vi "set settings from string.vi"(8 "error constant":errorcluster, 10 "String":string, 11 "VI in":refnum<vi>) -> (0 "error out":errorcluster)   [LabVIEW 2016, in "SaveLoad.lvlib"]
uses:
  SaveLoad.lvlib
  <vilib>/Utility/Data Type/Type Definitions/Data Type.ctl
  <vilib>/Utility/Data Type/NI_Data Type.lvlib
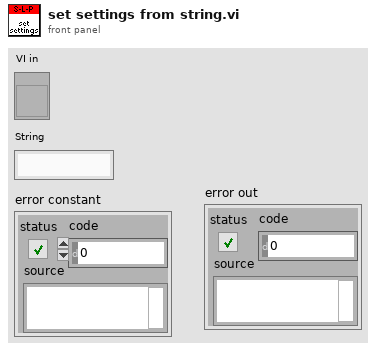
[diagram p1: front panel]
types:
  T1 = typedef "NI_Data Type.lvlib/Data Type.ctl" = enum8{"Invalid Type", "Void", "I8", "I16", "I32", "I64", "U8", "U16", "U32", "U64", "Single Float", "Double Float", "Extended Float", "Single Complex", "Double Complex", "Extended Complex", "Enum U8", "Enum U16", "Enum U32", "Enum U64", "Single Float With Unit", "Double Float With Unit", "Extended Float With Unit", "Single Complex with Unit", "Double Complex with Unit", "Extended Complex with Unit", "Boolean", "String", "Path", "Picture", "Tag", "Array", "Cluster", "Variant", "LV Variant", "Waveform", "Timestamp", "Digital Waveform", "Digital Data", "ExpressData", "Refnum", "External Data", "VI", "Poly VI", "LabVIEW Class Instance", "Fixed Point"}
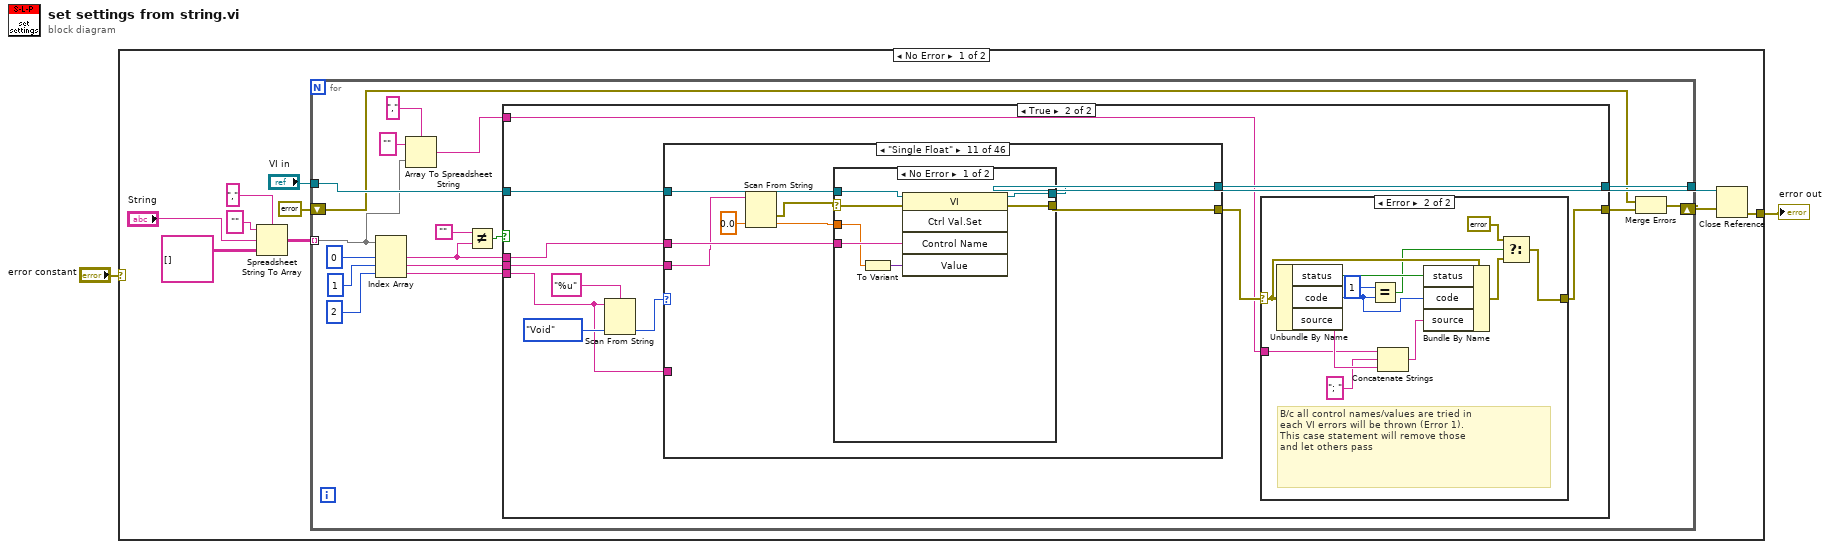
[diagram p0: block diagram]
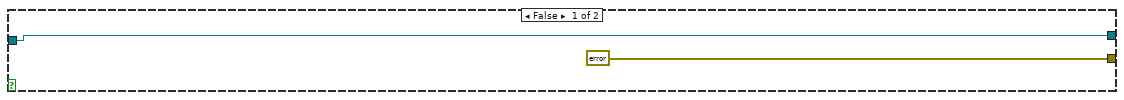
[diagram p2: hidden frame]
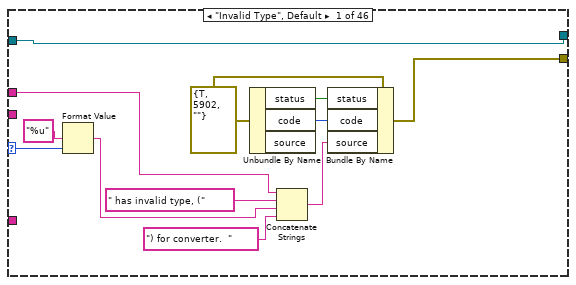
[diagram p4: hidden frame]
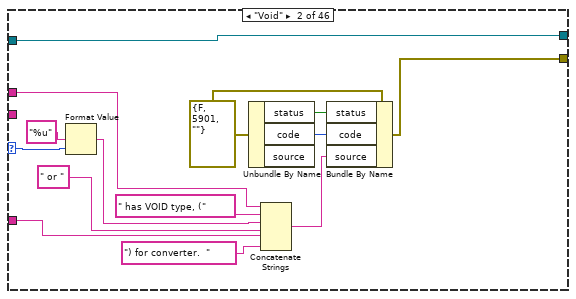
[diagram p5: hidden frame]
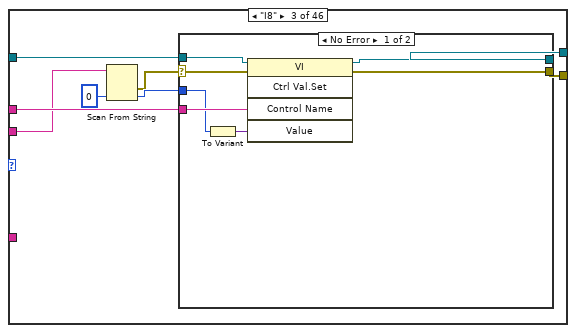
[diagram p6: hidden frame]
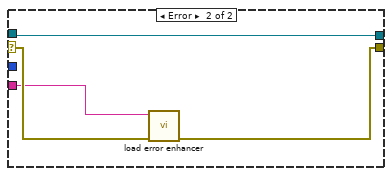
[diagram p7: hidden frame]
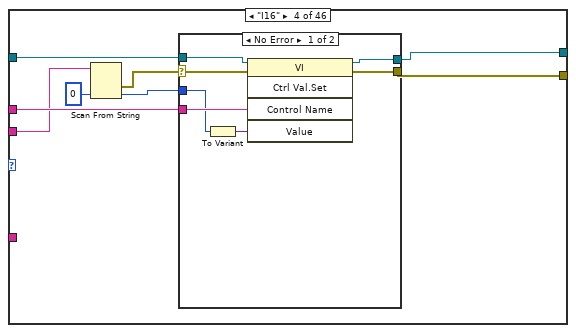
[diagram p8: hidden frame]
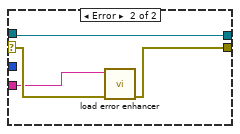
[diagram p9: hidden frame]
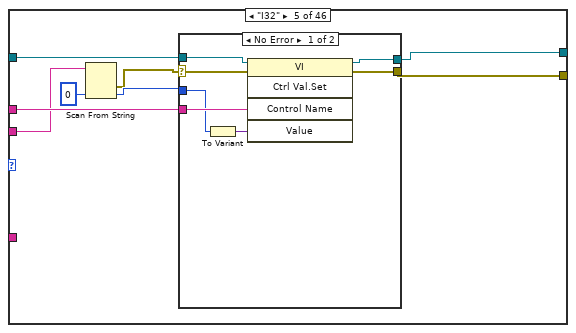
[diagram p10: hidden frame]
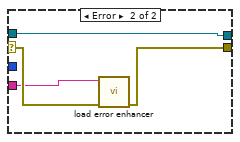
[diagram p11: hidden frame]
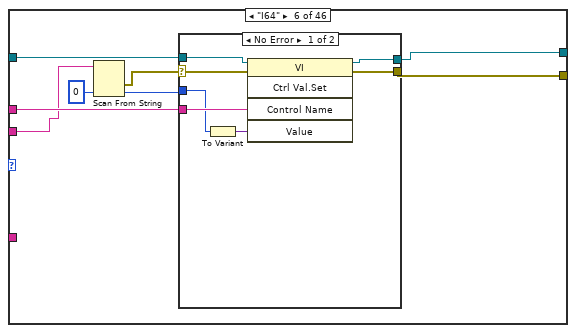
[diagram p12: hidden frame]
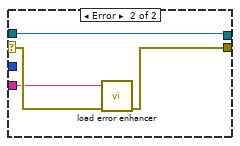
[diagram p13: hidden frame]
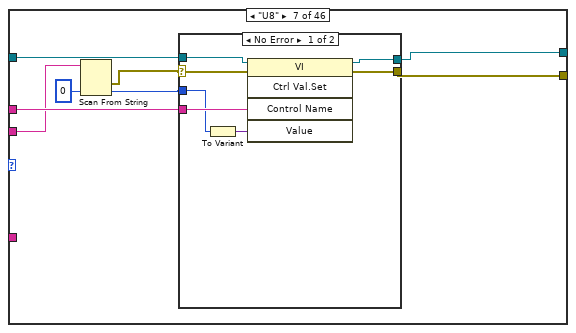
[diagram p14: hidden frame]
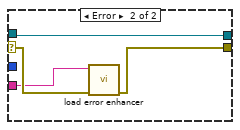
[diagram p15: hidden frame]
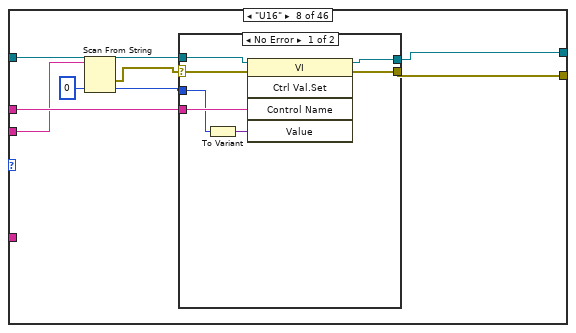
[diagram p16: hidden frame]
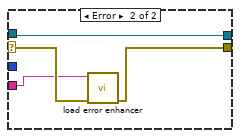
[diagram p17: hidden frame]
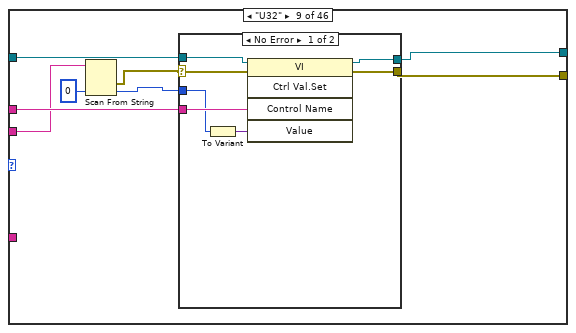
[diagram p18: hidden frame]
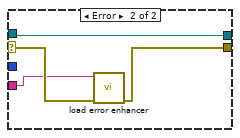
[diagram p19: hidden frame]
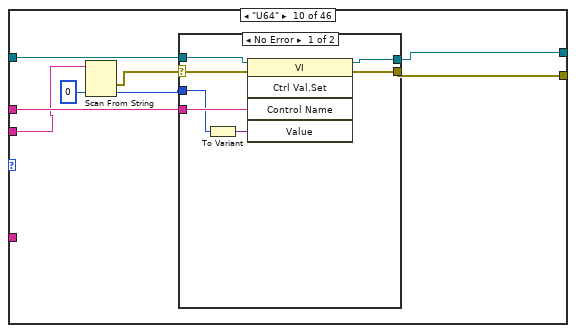
[diagram p20: hidden frame]
diagram:
  n1 = case shown="No Error" "error constant" {
    selector: "error constant" -> [_ w414]
    tunnel: [w12 w414] -> w2
    frame No Error {
      n2 = Spreadsheet String To Array(delimiter (Tab)=",", format string="", spreadsheet string="String", array type (2D Dbl)=string[][] []) -> (array=w8:string[][])
      n3 = for {
        tunnel: w8 -> [w16] mode=indexing
        tunnel: "VI in" -> [w25]
        tunnel: [w24] -> w10
        shift-right: [w21] -> w11
        shift-left: errorcluster {"status"=FALSE, "code"=0, "source"=""} ("error out") -> [w20]
        n4 = Index Array(array=w16, index #1=0 ("index"), index #2=1 ("index"), index #3=2 ("index")) -> (element #1=w18:string, element #2=w26:string, element #3=w22:string)
        n5 = Array To Spreadsheet String(delimiter (Tab)=",", array=w16, 3:"" ("format string")) -> (spreadsheet string=w13:string)
        n6 = Not Equal?(x="", y=w18) -> (x != y?=w17:bool)
        n7 = case shown="True" w17 {
          tunnel: w26 -> [_ w42]
          tunnel: w25 -> [w31 w41]
          tunnel: [w31 w40] -> w24
          tunnel: [errorcluster {"status"=FALSE, "code"=0, "source"=""} ("error out") w32] -> w23
          tunnel: w22 -> [_ w37]
          tunnel: w18 -> [_ w34]
          tunnel: w13 -> [_ w33]
          frame False {
          }
          frame True {
            n8 = Scan From String(format string="%u", input string=w37, default 1=Data_Type."Void" ("Type")) -> (output 1=w39:T1)  [unwired: 2 in, 3 out]
            n9 = case shown="\"Single Float\"" w39 {
              selector: w39 -> [w58 w72 _ _ _ _ _ _ _ _ _ _ _ _ _ _ _ _ _ _ _ _ _ _ _ _ _ _ _ _ _ _ _ _ _ _ _ _ _ _ _ _ _ _ _ _]
              tunnel: w34 -> [w62 w74 w89 w108 w127 w146 w165 w184 w203 w222 w241 w260 w279 w301 w318 w327 _ _ _ _ _ _ _ _ _ _ _ _ _ _ _ _ _ _ _ _ _ _ _ _ _ _ _ _ _ w402]
              tunnel: w42 -> [_ _ w82 w101 w120 w141 w160 w179 w196 w217 w236 w253 w272 w296 w317 w323 _ _ _ _ _ _ _ _ _ _ _ _ _ _ _ _ _ _ _ _ _ _ _ _ _ _ _ _ _ w398]
              tunnel: w41 -> [w67 w81 w88 w107 w126 w145 w164 w183 w202 w221 w240 w259 w278 w300 w316 w320 w338 w340 w342 w344 w346 w348 w350 w352 w354 w356 w358 w360 w362 w364 w366 w368 w370 w372 w374 w376 w378 w380 w382 w384 w386 w388 w390 w392 w394 w401]
              tunnel: [w67 w81 w87 w106 w125 w144 w163 w182 w201 w220 w239 w258 w277 w299 w315 w326 w338 w340 w342 w344 w346 w348 w350 w352 w354 w356 w358 w360 w362 w364 w366 w368 w370 w372 w374 w376 w378 w380 w382 w384 w386 w388 w390 w392 w394 w400] -> w40
              tunnel: [w65 w75 w86 w105 w124 w143 w162 w181 w200 w219 w238 w257 w276 w298 w314 w321 errorcluster {"status"=FALSE, "code"=0, "source"=""} ("error out") errorcluster {"status"=FALSE, "code"=0, "source"=""} ("error out") errorcluster {"status"=FALSE, "code"=0, "source"=""} ("error out") errorcluster {"status"=FALSE, "code"=0, "source"=""} ("error out") errorcluster {"status"=FALSE, "code"=0, "source"=""} ("error out") errorcluster {"status"=FALSE, "code"=0, "source"=""} ("error out") errorcluster {"status"=FALSE, "code"=0, "source"=""} ("error out") errorcluster {"status"=FALSE, "code"=0, "source"=""} ("error out") errorcluster {"status"=FALSE, "code"=0, "source"=""} ("error out") errorcluster {"status"=FALSE, "code"=0, "source"=""} ("error out") errorcluster {"status"=FALSE, "code"=0, "source"=""} ("error out") errorcluster {"status"=FALSE, "code"=0, "source"=""} ("error out") errorcluster {"status"=FALSE, "code"=0, "source"=""} ("error out") errorcluster {"status"=FALSE, "code"=0, "source"=""} ("error out") errorcluster {"status"=FALSE, "code"=0, "source"=""} ("error out") errorcluster {"status"=FALSE, "code"=0, "source"=""} ("error out") errorcluster {"status"=FALSE, "code"=0, "source"=""} ("error out") errorcluster {"status"=FALSE, "code"=0, "source"=""} ("error out") errorcluster {"status"=FALSE, "code"=0, "source"=""} ("error out") errorcluster {"status"=FALSE, "code"=0, "source"=""} ("error out") errorcluster {"status"=FALSE, "code"=0, "source"=""} ("error out") errorcluster {"status"=FALSE, "code"=0, "source"=""} ("error out") errorcluster {"status"=FALSE, "code"=0, "source"=""} ("error out") errorcluster {"status"=FALSE, "code"=0, "source"=""} ("error out") errorcluster {"status"=FALSE, "code"=0, "source"=""} ("error out") errorcluster {"status"=FALSE, "code"=0, "source"=""} ("error out") errorcluster {"status"=FALSE, "code"=0, "source"=""} ("error out") errorcluster {"status"=FALSE, "code"=0, "source"=""} ("error out") errorcluster {"status"=FALSE, "code"=0, "source"=""} ("error out") w399] -> w35
              tunnel: w37 -> [_ w70 _ _ _ _ _ _ _ _ _ _ _ _ _ _ _ _ _ _ _ _ _ _ _ _ _ _ _ _ _ _ _ _ _ _ _ _ _ _ _ _ _ _ _ _]
              frame "Invalid Type", Default {
                w66 = errorcluster {"status"=TRUE, "code"=5902, "source"=""} ("error constant")
                n10 = Format Value(format string="%u", value (0)=w58) -> (output string=w57:string)  [unwired: 1 in]
                n11 = Unbundle By Name(w66) -> ("status"=w64:bool, "code"=w63:i32)  [unwired: 1 out]
                n12 = Concatenate Strings(w62, " has invalid type, (", w57, ") for converter.  " ("string")) -> (w60:string)
                n13 = Bundle By Name(cluster=w66, "status"=w64, "code"=w63, "source"=w60) -> (w65:errorcluster)
              }
              frame "Void" {
                w80 = errorcluster {"status"=FALSE, "code"=5901, "source"=""} ("error constant")
                n14 = Format Value(format string="%u", value (0)=w72) -> (output string=w69:string)  [unwired: 1 in]
                n15 = Unbundle By Name(w80) -> ("status"=w79:bool, "code"=w78:i32)  [unwired: 1 out]
                n16 = Concatenate Strings(w74, " has VOID type, (", w69, " or " ("string"), w70, ") for converter.  " ("string")) -> (w76:string)
                n17 = Bundle By Name(cluster=w80, "status"=w79, "code"=w78, "source"=w76) -> (w75:errorcluster)
              }
              frame "I8" {
                n18 = Scan From String(input string=w82, default 1=i8 0 ("default value 1")) -> (error out=w84:errorcluster, output 1=w85:i8)  [unwired: 3 in, 2 out]
                n19 = case shown="No Error" w84 {
                  selector: w84 -> [w90 w98]
                  tunnel: [w96 w100] -> w87
                  tunnel: [w95 w99] -> w86
                  tunnel: w89 -> [w94 w97]
                  tunnel: w85 -> [w92 _]
                  tunnel: w88 -> [w91 w100]
                  frame No Error {
                    n20 = To Variant(anything=w92) -> (Variant=w93:variant)
                    n21 = invoke class="VI" method="Ctrl Val.Set"(reference=w91, error in=w90, "Control Name"=w94, "Value"=w93) -> (reference out=w96:refnum<vi>, error out=w95:errorcluster)  [unwired: 1 in, 3 out]
                  }
                  frame Error {
                    n22 = call "load error enhancer.vi"("error in (no error)"=w98, "format string"=w97) -> ("error out"=w99:errorcluster)  [unwired: 9 in]
                  }
                }
              }
              frame "I16" {
                n23 = Scan From String(input string=w101, default 1=i16 0 ("default value 1")) -> (error out=w104:errorcluster, output 1=w103:i16)  [unwired: 3 in, 2 out]
                n24 = case shown="No Error" w104 {
                  selector: w104 -> [w109 w118]
                  tunnel: [w115 w119] -> w106
                  tunnel: [w114 w116] -> w105
                  tunnel: w108 -> [w113 w117]
                  tunnel: w103 -> [w111 _]
                  tunnel: w107 -> [w110 w119]
                  frame No Error {
                    n25 = To Variant(anything=w111) -> (Variant=w112:variant)
                    n26 = invoke class="VI" method="Ctrl Val.Set"(reference=w110, error in=w109, "Control Name"=w113, "Value"=w112) -> (reference out=w115:refnum<vi>, error out=w114:errorcluster)  [unwired: 1 in, 3 out]
                  }
                  frame Error {
                    n27 = call "load error enhancer.vi"("error in (no error)"=w118, "format string"=w117) -> ("error out"=w116:errorcluster)  [unwired: 9 in]
                  }
                }
              }
              frame "I32" {
                n28 = Scan From String(input string=w120, default 1=0 ("default value 1")) -> (error out=w121:errorcluster, output 1=w122:i32)  [unwired: 3 in, 2 out]
                n29 = case shown="No Error" w121 {
                  selector: w121 -> [w128 w137]
                  tunnel: [w134 w138] -> w125
                  tunnel: [w133 w135] -> w124
                  tunnel: w127 -> [w132 w136]
                  tunnel: w122 -> [w130 _]
                  tunnel: w126 -> [w129 w138]
                  frame No Error {
                    n30 = To Variant(anything=w130) -> (Variant=w131:variant)
                    n31 = invoke class="VI" method="Ctrl Val.Set"(reference=w129, error in=w128, "Control Name"=w132, "Value"=w131) -> (reference out=w134:refnum<vi>, error out=w133:errorcluster)  [unwired: 1 in, 3 out]
                  }
                  frame Error {
                    n32 = call "load error enhancer.vi"("error in (no error)"=w137, "format string"=w136) -> ("error out"=w135:errorcluster)  [unwired: 9 in]
                  }
                }
              }
              frame "I64" {
                n33 = Scan From String(input string=w141, default 1=i64 0 ("default value 1")) -> (error out=w139:errorcluster, output 1=w140:i64)  [unwired: 3 in, 2 out]
                n34 = case shown="No Error" w139 {
                  selector: w139 -> [w147 w155]
                  tunnel: [w153 w156] -> w144
                  tunnel: [w152 w157] -> w143
                  tunnel: w146 -> [w151 w154]
                  tunnel: w140 -> [w149 _]
                  tunnel: w145 -> [w148 w156]
                  frame No Error {
                    n35 = To Variant(anything=w149) -> (Variant=w150:variant)
                    n36 = invoke class="VI" method="Ctrl Val.Set"(reference=w148, error in=w147, "Control Name"=w151, "Value"=w150) -> (reference out=w153:refnum<vi>, error out=w152:errorcluster)  [unwired: 1 in, 3 out]
                  }
                  frame Error {
                    n37 = call "load error enhancer.vi"("error in (no error)"=w155, "format string"=w154) -> ("error out"=w157:errorcluster)  [unwired: 9 in]
                  }
                }
              }
              frame "U8" {
                n38 = Scan From String(input string=w160, default 1=u8 0 ("default value 1")) -> (error out=w158:errorcluster, output 1=w159:u8)  [unwired: 3 in, 2 out]
                n39 = case shown="No Error" w158 {
                  selector: w158 -> [w166 w174]
                  tunnel: [w172 w175] -> w163
                  tunnel: [w171 w176] -> w162
                  tunnel: w165 -> [w170 w173]
                  tunnel: w159 -> [w168 _]
                  tunnel: w164 -> [w167 w175]
                  frame No Error {
                    n40 = To Variant(anything=w168) -> (Variant=w169:variant)
                    n41 = invoke class="VI" method="Ctrl Val.Set"(reference=w167, error in=w166, "Control Name"=w170, "Value"=w169) -> (reference out=w172:refnum<vi>, error out=w171:errorcluster)  [unwired: 1 in, 3 out]
                  }
                  frame Error {
                    n42 = call "load error enhancer.vi"("error in (no error)"=w174, "format string"=w173) -> ("error out"=w176:errorcluster)  [unwired: 9 in]
                  }
                }
              }
              frame "U16" {
                n43 = Scan From String(input string=w179, default 1=u16 0 ("default value 1")) -> (error out=w177:errorcluster, output 1=w178:u16)  [unwired: 3 in, 2 out]
                n44 = case shown="No Error" w177 {
                  selector: w177 -> [w185 w193]
                  tunnel: [w191 w194] -> w182
                  tunnel: [w190 w195] -> w181
                  tunnel: w184 -> [w189 w192]
                  tunnel: w178 -> [w187 _]
                  tunnel: w183 -> [w186 w194]
                  frame No Error {
                    n45 = To Variant(anything=w187) -> (Variant=w188:variant)
                    n46 = invoke class="VI" method="Ctrl Val.Set"(reference=w186, error in=w185, "Control Name"=w189, "Value"=w188) -> (reference out=w191:refnum<vi>, error out=w190:errorcluster)  [unwired: 1 in, 3 out]
                  }
                  frame Error {
                    n47 = call "load error enhancer.vi"("error in (no error)"=w193, "format string"=w192) -> ("error out"=w195:errorcluster)  [unwired: 9 in]
                  }
                }
              }
              frame "U32" {
                n48 = Scan From String(input string=w196, default 1=u32 0 ("default value 1")) -> (error out=w197:errorcluster, output 1=w198:u32)  [unwired: 3 in, 2 out]
                n49 = case shown="No Error" w197 {
                  selector: w197 -> [w204 w212]
                  tunnel: [w210 w213] -> w201
                  tunnel: [w209 w214] -> w200
                  tunnel: w203 -> [w208 w211]
                  tunnel: w198 -> [w206 _]
                  tunnel: w202 -> [w205 w213]
                  frame No Error {
                    n50 = To Variant(anything=w206) -> (Variant=w207:variant)
                    n51 = invoke class="VI" method="Ctrl Val.Set"(reference=w205, error in=w204, "Control Name"=w208, "Value"=w207) -> (reference out=w210:refnum<vi>, error out=w209:errorcluster)  [unwired: 1 in, 3 out]
                  }
                  frame Error {
                    n52 = call "load error enhancer.vi"("error in (no error)"=w212, "format string"=w211) -> ("error out"=w214:errorcluster)  [unwired: 9 in]
                  }
                }
              }
              frame "U64" {
                n53 = Scan From String(input string=w217, default 1=u64 0 ("default value 1")) -> (error out=w215:errorcluster, output 1=w216:u64)  [unwired: 3 in, 2 out]
                n54 = case shown="No Error" w215 {
                  selector: w215 -> [w223 w231]
                  tunnel: [w229 w232] -> w220
                  tunnel: [w228 w233] -> w219
                  tunnel: w222 -> [w227 w230]
                  tunnel: w216 -> [w225 _]
                  tunnel: w221 -> [w224 w232]
                  frame No Error {
                    n55 = To Variant(anything=w225) -> (Variant=w226:variant)
                    n56 = invoke class="VI" method="Ctrl Val.Set"(reference=w224, error in=w223, "Control Name"=w227, "Value"=w226) -> (reference out=w229:refnum<vi>, error out=w228:errorcluster)  [unwired: 1 in, 3 out]
                  }
                  frame Error {
                    n57 = call "load error enhancer.vi"("error in (no error)"=w231, "format string"=w230) -> ("error out"=w233:errorcluster)  [unwired: 9 in]
                  }
                }
              }
              frame "Single Float" {
                n58 = Scan From String(input string=w236, default 1=sgl 0.0 ("default value 1")) -> (error out=w234:errorcluster, output 1=w235:sgl)  [unwired: 3 in, 2 out]
                n59 = case shown="No Error" w234 {
                  selector: w234 -> [w242 w250]
                  tunnel: [w248 w251] -> w239
                  tunnel: [w247 w252] -> w238
                  tunnel: w241 -> [w246 w249]
                  tunnel: w235 -> [w244 _]
                  tunnel: w240 -> [w243 w251]
                  frame No Error {
                    n60 = To Variant(anything=w244) -> (Variant=w245:variant)
                    n61 = invoke class="VI" method="Ctrl Val.Set"(reference=w243, error in=w242, "Control Name"=w246, "Value"=w245) -> (reference out=w248:refnum<vi>, error out=w247:errorcluster)  [unwired: 1 in, 3 out]
                  }
                  frame Error {
                    n62 = call "load error enhancer.vi"("error in (no error)"=w250, "format string"=w249) -> ("error out"=w252:errorcluster)  [unwired: 9 in]
                  }
                }
              }
              frame "Double Float" {
                n63 = Scan From String(input string=w253, default 1=0.0 ("default value 1")) -> (error out=w255:errorcluster, output 1=w254:dbl)  [unwired: 3 in, 2 out]
                n64 = case shown="No Error" w255 {
                  selector: w255 -> [w261 w269]
                  tunnel: [w267 w268] -> w258
                  tunnel: [w266 w271] -> w257
                  tunnel: w260 -> [w265 w270]
                  tunnel: w254 -> [w263 _]
                  tunnel: w259 -> [w262 w268]
                  frame No Error {
                    n65 = To Variant(anything=w263) -> (Variant=w264:variant)
                    n66 = invoke class="VI" method="Ctrl Val.Set"(reference=w262, error in=w261, "Control Name"=w265, "Value"=w264) -> (reference out=w267:refnum<vi>, error out=w266:errorcluster)  [unwired: 1 in, 3 out]
                  }
                  frame Error {
                    n67 = call "load error enhancer.vi"("error in (no error)"=w269, "format string"=w270) -> ("error out"=w271:errorcluster)  [unwired: 9 in]
                  }
                }
              }
              frame "Extended Float" {
                n68 = Scan From String(input string=w272, default 1=ext 0.0 ("default value 1")) -> (error out=w274:errorcluster, output 1=w273:ext)  [unwired: 3 in, 2 out]
                n69 = case shown="No Error" w274 {
                  selector: w274 -> [w280 w288]
                  tunnel: [w286 w289] -> w277
                  tunnel: [w285 w290] -> w276
                  tunnel: w279 -> [w284 w287]
                  tunnel: w273 -> [w282 _]
                  tunnel: w278 -> [w281 w289]
                  frame No Error {
                    n70 = To Variant(anything=w282) -> (Variant=w283:variant)
                    n71 = invoke class="VI" method="Ctrl Val.Set"(reference=w281, error in=w280, "Control Name"=w284, "Value"=w283) -> (reference out=w286:refnum<vi>, error out=w285:errorcluster)  [unwired: 1 in, 3 out]
                  }
                  frame Error {
                    n72 = call "load error enhancer.vi"("error in (no error)"=w288, "format string"=w287) -> ("error out"=w290:errorcluster)  [unwired: 9 in]
                  }
                }
              }
              frame "Boolean" {
                n73 = Scan From String(input string=w296, default 1=i8 0 ("default value 1")) -> (error out=w295:errorcluster, output 1=w294:i8)  [unwired: 3 in, 2 out]
                n74 = Number To Boolean Array(number=w294) -> (Boolean array=w293:bool[])
                n75 = Index Array(array=w293, index=0) -> (element=w292:bool)
                n76 = case shown="No Error" w295 {
                  selector: w295 -> [w303 w310]
                  tunnel: [w308 w311] -> w299
                  tunnel: [w307 w312] -> w298
                  tunnel: w301 -> [w306 w309]
                  tunnel: w292 -> [w302 _]
                  tunnel: w300 -> [w304 w311]
                  frame No Error {
                    n77 = To Variant(anything=w302) -> (Variant=w305:variant)
                    n78 = invoke class="VI" method="Ctrl Val.Set"(reference=w304, error in=w303, "Control Name"=w306, "Value"=w305) -> (reference out=w308:refnum<vi>, error out=w307:errorcluster)  [unwired: 1 in, 3 out]
                  }
                  frame Error {
                    n79 = call "load error enhancer.vi"("error in (no error)"=w310, "format string"=w309) -> ("error out"=w312:errorcluster)  [unwired: 9 in]
                  }
                }
              }
              frame "String" {
                n80 = To Variant(anything=w317) -> (Variant=w313:variant)
                n81 = invoke class="VI" method="Ctrl Val.Set"(reference=w316, "Control Name"=w318, "Value"=w313) -> (reference out=w315:refnum<vi>, error out=w314:errorcluster)  [unwired: 2 in, 3 out]
              }
              frame "Path" {
                n82 = call <vilib>:"Trim Whitespace.vi"("string"=w323) -> ("trimmed string"=w319:string)  [unwired: 1 in]
                n83 = String To Path(string=w319) -> (path=w325:path)
                n84 = To Variant(anything=w325) -> (Variant=w324:variant)
                n85 = invoke class="VI" method="Ctrl Val.Set"(reference=w320, "Control Name"=w327, "Value"=w324) -> (reference out=w326:refnum<vi>, error out=w322:errorcluster)  [unwired: 2 in, 3 out]
                n86 = case shown="Error" w322 {
                  selector: w322 -> [w328 w336]
                  tunnel: [w328 w335] -> w321
                  tunnel: w319 -> [_ w330]
                  frame No Error {
                  }
                  frame Error {
                    n87 = Unbundle By Name(w336) -> ("status"=w334:bool, "code"=w333:i32, "source"=w331:string)
                    n88 = Concatenate Strings(w330, "; " ("string"), w331) -> (w332:string)
                    n89 = Bundle By Name(cluster=w336, "status"=w334, "code"=w333, "source"=w332) -> (w335:errorcluster)
                  }
                }
              }
              frame "Cluster" {
              }
              frame "Variant" {
              }
              frame "LV Variant" {
              }
              frame "Waveform" {
              }
              frame "Timestamp" {
              }
              frame "Digital Waveform" {
              }
              frame "Digital Data" {
              }
              frame "ExpressData" {
              }
              frame "Refnum" {
              }
              frame "External Data" {
              }
              frame "VI" {
              }
              frame "Poly VI" {
              }
              frame "LabVIEW Class Instance" {
              }
              frame "Single Complex" {
              }
              frame "Double Complex" {
              }
              frame "Extended Complex" {
              }
              frame "Enum U64" {
              }
              frame "Enum U8" {
              }
              frame "Enum U16" {
              }
              frame "Enum U32" {
              }
              frame "Single Float With Unit" {
              }
              frame "Double Float With Unit" {
              }
              frame "Extended Float With Unit" {
              }
              frame "Single Complex with Unit" {
              }
              frame "Double Complex with Unit" {
              }
              frame "Extended Complex with Unit" {
              }
              frame "Picture" {
              }
              frame "Tag" {
              }
              frame "Array" {
              }
              frame "Fixed Point" {
                n90 = Scan From String(input string=w398, default 1=fxp<+,1,1> 0.0 ("default value 1")) -> (error out=w397:errorcluster, output 1=w395:dbl)  [unwired: 3 in, 2 out]
                n91 = case shown="No Error" w397 {
                  selector: w397 -> [w403 w411]
                  tunnel: [w409 w412] -> w400
                  tunnel: [w408 w413] -> w399
                  tunnel: w402 -> [w407 w410]
                  tunnel: w395 -> [w405 _]
                  tunnel: w401 -> [w404 w412]
                  frame No Error {
                    n92 = To Variant(anything=w405) -> (Variant=w406:variant)
                    n93 = invoke class="VI" method="Ctrl Val.Set"(reference=w404, error in=w403, "Control Name"=w407, "Value"=w406) -> (reference out=w409:refnum<vi>, error out=w408:errorcluster)  [unwired: 1 in, 3 out]
                  }
                  frame Error {
                    n94 = call "load error enhancer.vi"("error in (no error)"=w411, "format string"=w410) -> ("error out"=w413:errorcluster)  [unwired: 9 in]
                  }
                }
              }
            }
            n95 = case shown="Error" w35 {
              selector: w35 -> [w43 w55]
              tunnel: [w43 w45] -> w32
              tunnel: w33 -> [_ w51]
              frame No Error {
              }
              frame Error {
                # "B/c all control names/values are tried in \neach VI errors will be thrown (Error 1).  \nThis case statement will remove those \nand let others pass"
                n96 = Unbundle By Name(w55) -> ("status"=w54:bool, "code"=w48:i32, "source"=w52:string)
                n97 = Equal?(x=1, y=w48) -> (x = y?=w44:bool)
                n98 = Concatenate Strings(w51, "; " ("string"), w52) -> (w53:string)
                n99 = Bundle By Name(cluster=w55, "status"=w54, "code"=w48, "source"=w53) -> (w46:errorcluster)
                n100 = Select(t=errorcluster {"status"=FALSE, "code"=0, "source"=""} ("error constant"), s=w44, f=w46) -> (s? t:f=w45:errorcluster)
              }
            }
          }
        }
        n101 = Merge Errors(w20, w23) -> (w21:errorcluster)
      }
      n102 = Close Reference(reference=w10, error in (no error)=w11) -> (error out=w12:errorcluster)
    }
    frame Error {
    }
  }
  "error out" <- w2
